vi "Filter Present Satellites.vi"(11 "Satellites":T1[](array[typedef])) -> (3 "Filtered Satellites":T1[](array[typedef]))   [LabVIEW 2012, in "nmea.lvlib" / "nmea.lvclass"]
uses:
  nmea.lvclass
  Satellite.ctl
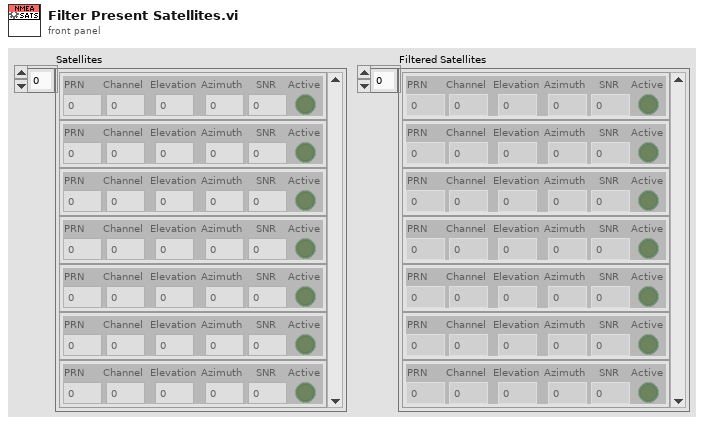
[diagram p1: front panel]
types:
  T1 = typedef "nmea.lvlib/nmea.lvclass/Satellite.ctl" = cluster{"PRN":u8, "Channel":u8, "Elevation":u8, "Azimuth":u16, "SNR":u8, "Active":bool}
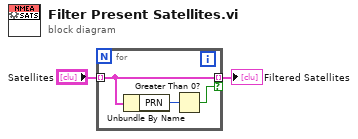
[diagram p0: block diagram]
diagram:
  n1 = for {
    tunnel: "Satellites" -> [w5] mode=indexing
    tunnel: [w5] -> w1 mode=indexing if=w3
    n2 = Unbundle By Name(w5) -> ("PRN"=w4:u8)
    n3 = Greater Than 0?(x=w4) -> (x > 0?=w3:bool)
  }
  "Filtered Satellites" <- w1
